vi "run conventional acq.vi"(8 "error in (no error)":errorcluster, 11 "Channel in":refnum<class "SPARC4_Channel.lvclass">) -> (0 "error out":errorcluster, 3 "Channel out":refnum<class "SPARC4_Channel.lvclass">)   [LabVIEW 2018, in "SPARC4_Channel.lvclass"]
doc: "Run the channel"
uses:
  SPARC4_Channel.lvclass
  C:/Users/Denis/Desktop/S4ACS/S4ACS/Channel/Channel.lvclass
  SPARC4_Channel.lvclass/SPARC4_Channel.ctl
  Channel/Channel.lvclass/Channel.ctl
  Sim_Ixon_Ultra/Sim_Ixon_Ultra.lvclass
  C:/Users/Denis/Desktop/S4ACS/S4ACS/Sim_CCD/Sim_CCD.lvclass
  State Machine/State Machine.lvclass
  Sim_CCD/Sim_CCD.lvclass
  RxTx/RxTx.lvclass
  Server/Server.lvclass
  Channel/Channel.lvclass
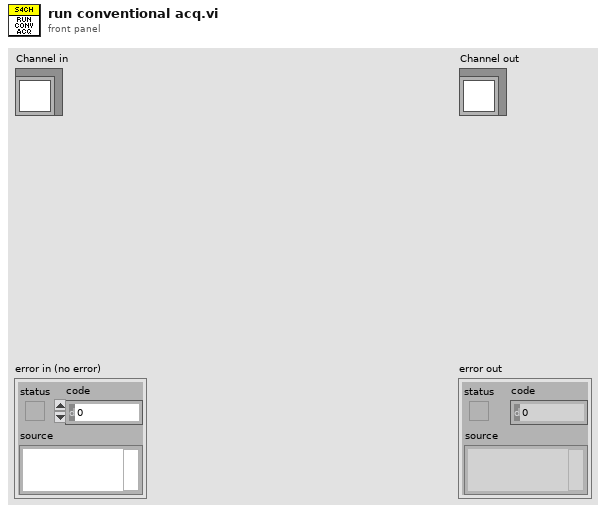
[diagram p1: front panel]
types:
  T1 = cluster{"State Machine.lvclass":refnum<class "State Machine.lvclass">, "RxTx.lvclass":refnum<class "RxTx.lvclass">, "Save_Header_RxTx.lvclass":refnum<class "RxTx.lvclass">, "Status SM.lvclass":refnum<class "State Machine.lvclass">, "Status RxTx.lvclass":refnum<class "RxTx.lvclass">, "servers array":refnum<class "Server.lvclass">[], "Events log file.lvclass":refnum<class "Log File.lvclass">, "Errors log file.lvclass":refnum<class "Log File.lvclass">, "Keywords log file.lvclass":refnum<class "Log File.lvclass">, "Sim_CCD.lvclass":refnum<class "Sim_CCD.lvclass">}
  T2 = typedef "LVDateTimeRec.ctl" = cluster{"fractional second":dbl, "second":i32, "minute":i32, "hour":i32, "day of month":i32, "month":i32, "year":i32, "day of week":i32, "day of year":i32, "DST":i32}
  T3 = cluster{"Time Acq Started":u32, "Image delay":u64, "Last update - CCD config":timestamp, "SYSTEMTIME":T2, "Readout time":dbl, "Time acq finished":u32, "effective exptime":dbl}
  T4 = cluster{"FRAMES_DONE":u16, "CCD_STATUS":string, "CURRENT_TEMPERATURE":i16, "TEMPERATURE_STATUS":string, "FRAME_EXPOSURE_TIME":dbl, "SERIAL_NUMBER":u16, "ACQUIRING":bool, "POWER":bool, "ACS MODE":bool}
  T5 = cluster{"Stop Acquisition":bool, "Abort Acquisition":bool, "Pause acquisition":bool, "wait expose command":bool, "video mode":bool, "stop app":bool}
  T6 = cluster{"CYCLES_DONE":u16, "LAST_IMAGE_NAME":string, "USED_DISK_SPACE":u16, "IMAGE_INDEX":u32, "acquisition error":bool}
  T7 = cluster{"EXPTIME":dbl, "#FRAMES":u32, "COOLER_POWER_STATUS":u16, "TEMP":i32}
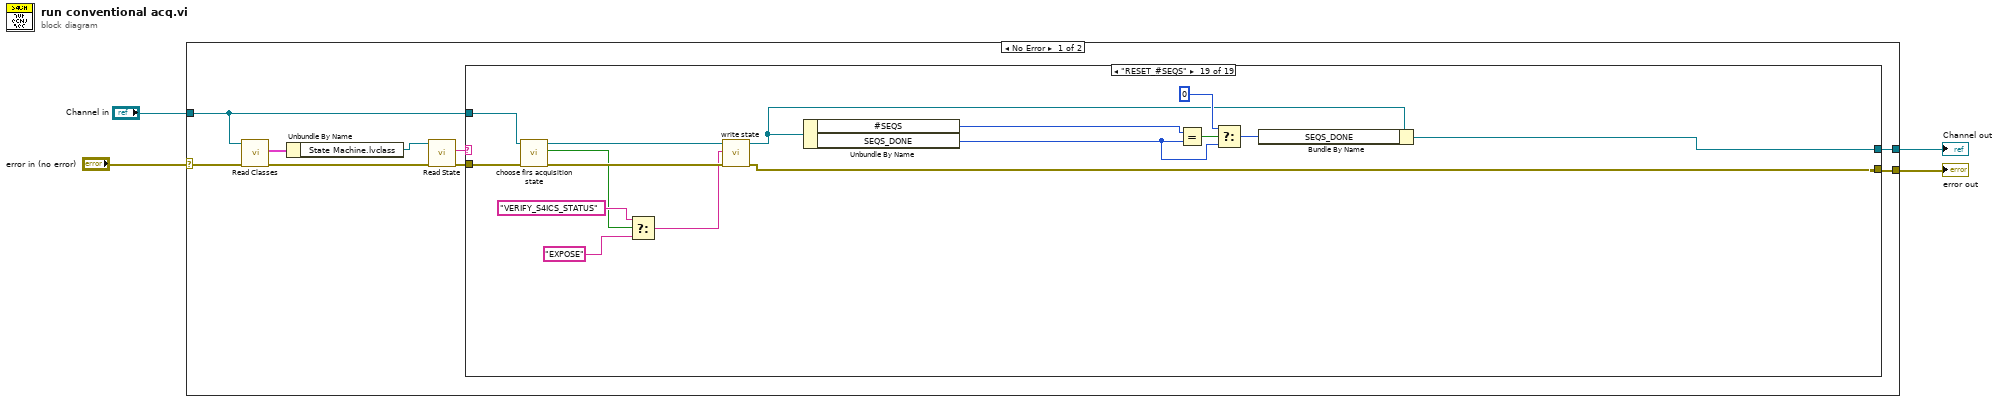
[diagram p0: block diagram]
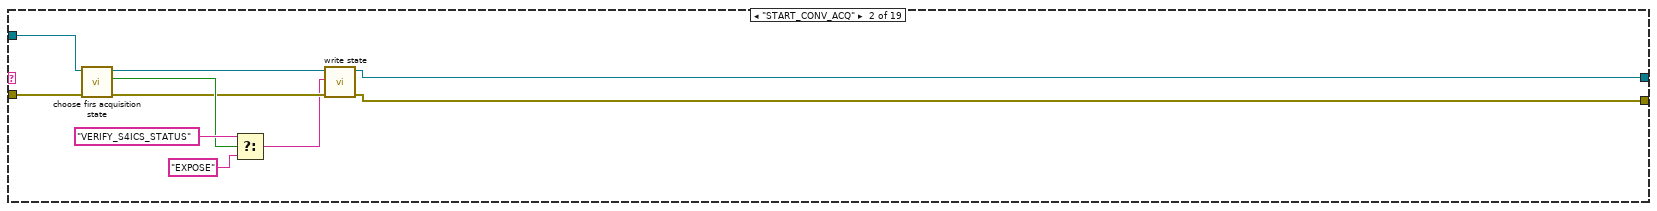
[diagram p3: hidden frame]
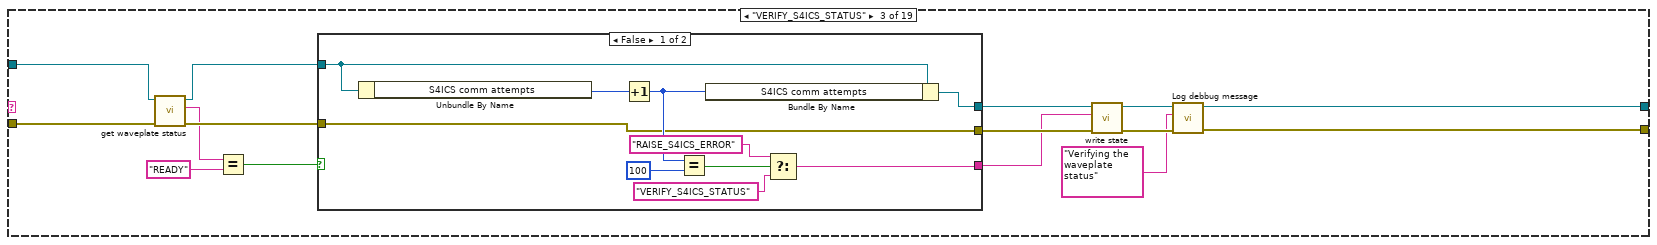
[diagram p4: hidden frame]
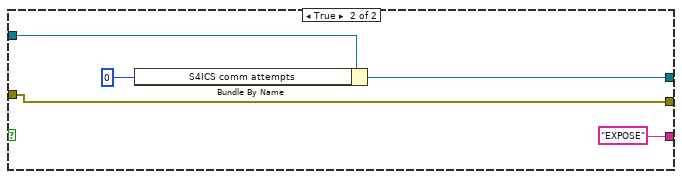
[diagram p5: hidden frame]
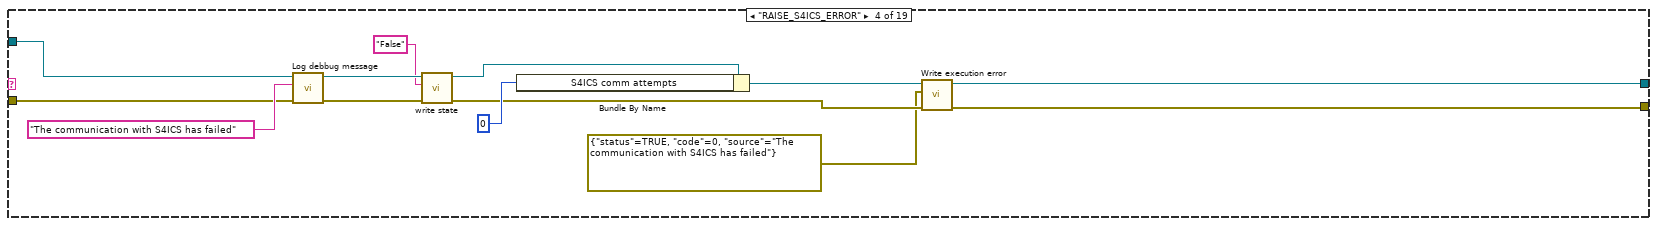
[diagram p6: hidden frame]
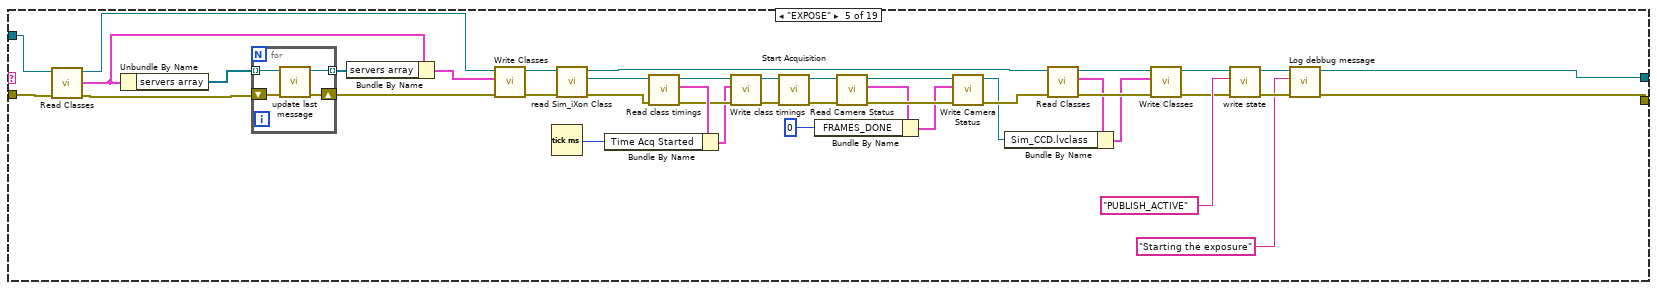
[diagram p7: hidden frame]
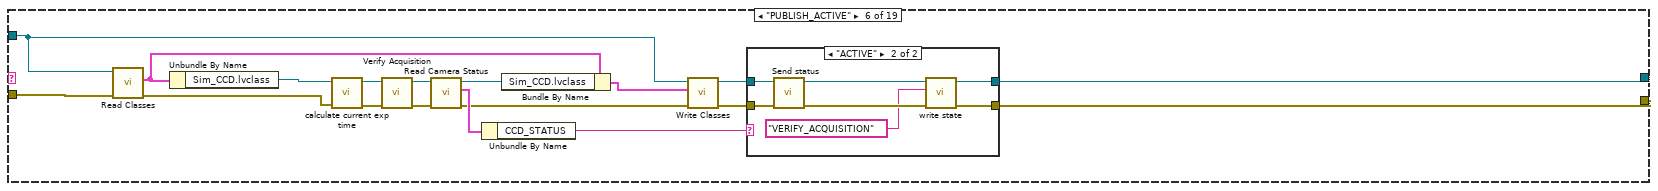
[diagram p8: hidden frame]
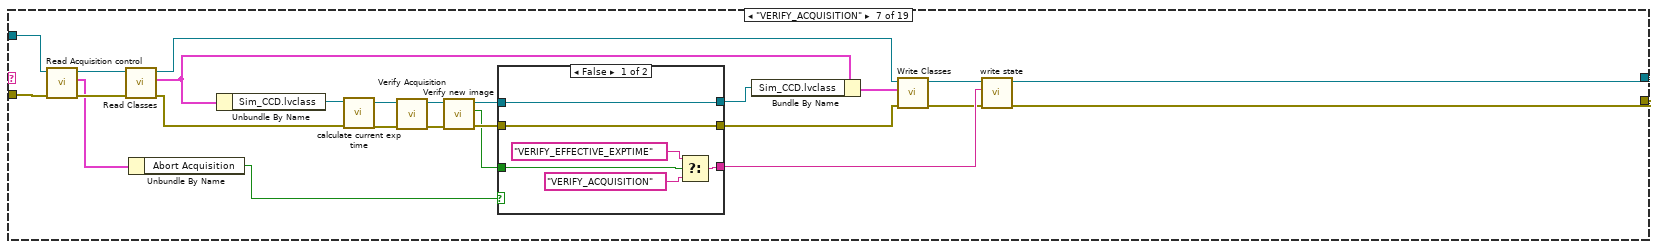
[diagram p10: hidden frame]
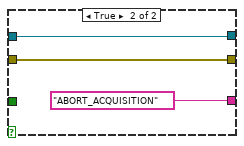
[diagram p11: hidden frame]
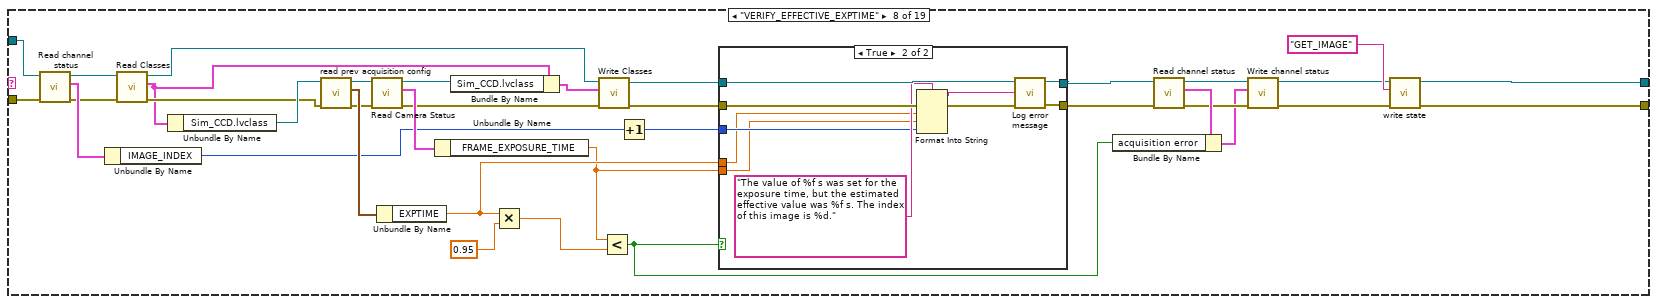
[diagram p12: hidden frame]
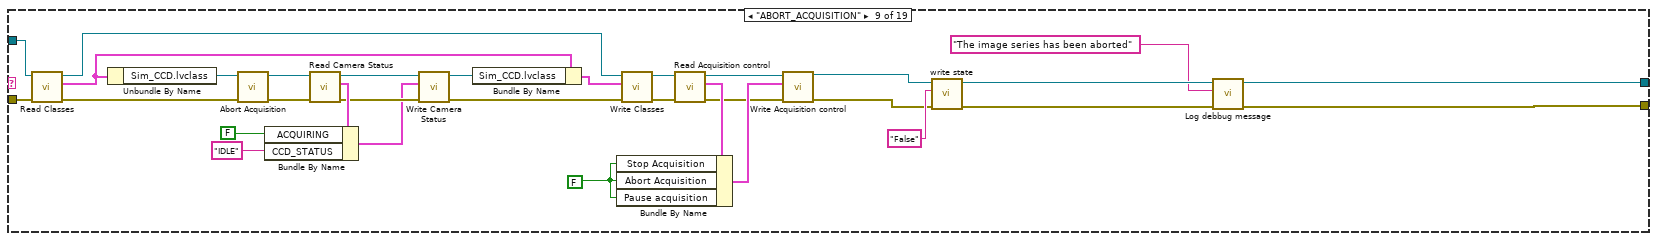
[diagram p14: hidden frame]
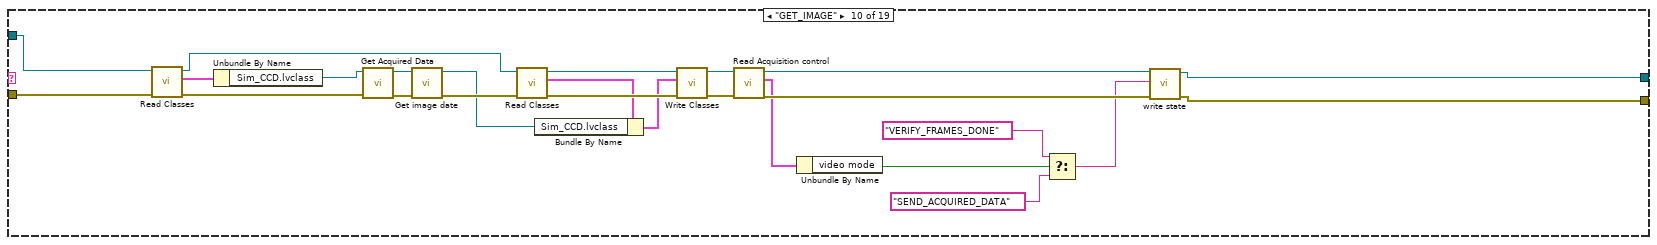
[diagram p15: hidden frame]
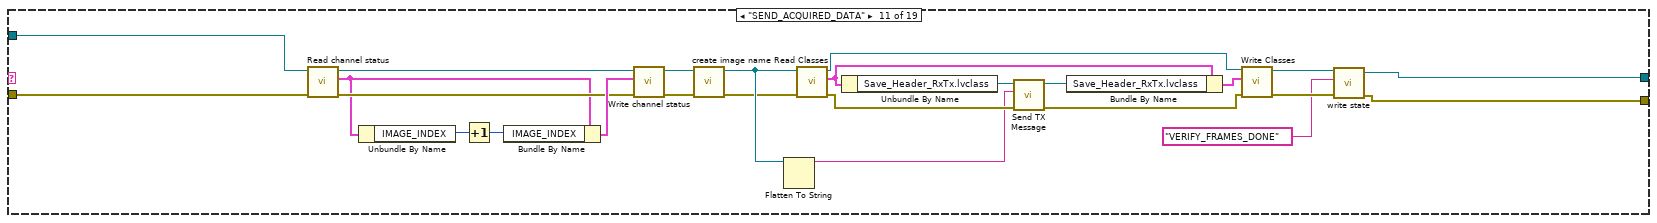
[diagram p16: hidden frame]
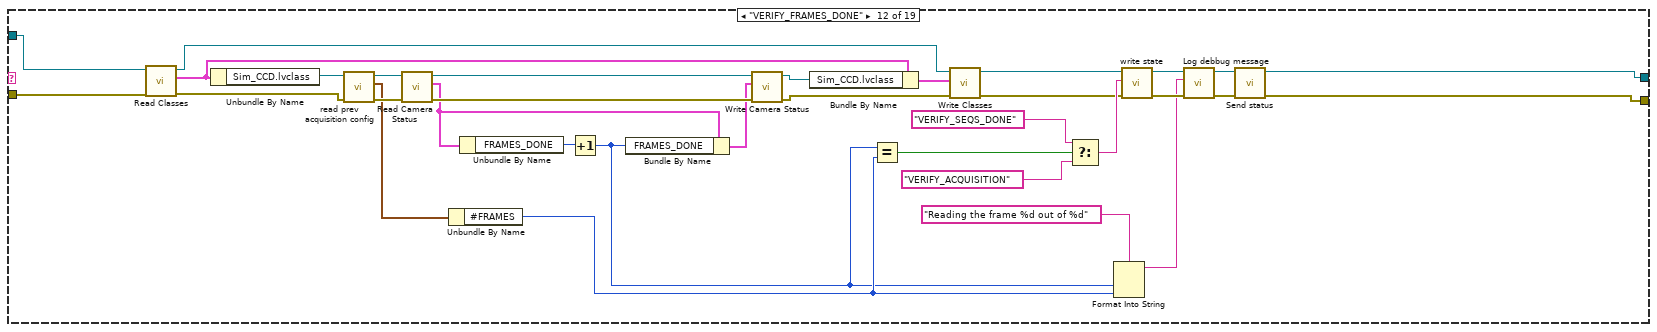
[diagram p17: hidden frame]
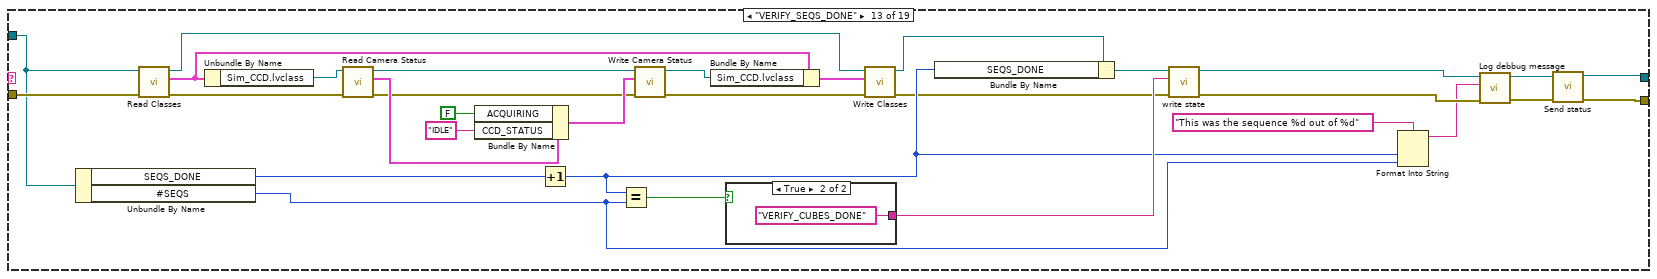
[diagram p18: hidden frame]
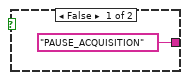
[diagram p19: hidden frame]
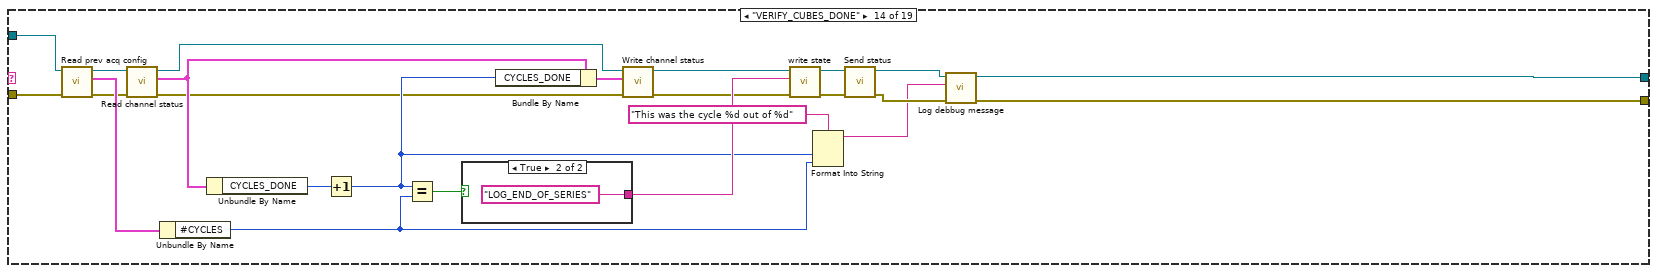
[diagram p20: hidden frame]
diagram:
  n1 = case shown="No Error" "error in (no error)" {
    selector: "error in (no error)" -> [w7 w486]
    tunnel: [w13 w486] -> w3
    tunnel: [w12 w485] -> w1
    tunnel: "Channel in" -> [w8 w485]
    frame No Error {
      n2 = call-dynamic "Read Classes.vi"("error in (no error)"=w7, "Channel in"=w8) -> ("error out"=w6:errorcluster, "Classes"=w9:T1)  [unwired: 7 in, 1 out]
      n3 = Unbundle By Name(w9) -> ("State Machine.lvclass"=w5:refnum<class "State Machine.lvclass">)
      n4 = call-dynamic "Read State.vi"("error in (no error)"=w6, "State Machine in"=w5) -> ("error out"=w11:errorcluster, "State"=w10:string)  [unwired: 7 in, 1 out]
      n5 = case shown="\"RESET_#SEQS\"" w10 {
        tunnel: w11 -> [w14 w22 w28 w66 w90 w124 w147 w188 w241 w275 w284 w328 w353 w378 w404 w408 w435 w460 w479]
        tunnel: [w14 w17 w34 w57 w100 w131 w163 w210 w244 w266 w304 w327 w340 w390 w400 w414 w438 w466 w481] -> w13
        tunnel: [w15 w18 w35 w58 w101 w132 w164 w211 w245 w265 w305 w326 w341 w389 w401 w413 w439 w465 w480] -> w12
        tunnel: w8 -> [w15 w21 w30 w67 w89 w119 w145 w182 w240 w276 w285 w329 w349 w376 w405 w409 w436 w461 w478]
        frame "False", Default {
        }
        frame "START_CONV_ACQ" {
          n6 = call "choose firs acquisition state.vi"("error in (no error)"=w22, "Channel in"=w21) -> ("error out"=w20:errorcluster, "verify S4ICS status"=w23:bool, "Channel out"=w19:refnum<class "SPARC4_Channel.lvclass">)  [unwired: 7 in]
          n7 = Select(t="VERIFY_S4ICS_STATUS" ("x"), s=w23, f="EXPOSE" ("x")) -> (s? t:f=w16:string)
          n8 = call "write state.vi"("error in (no error)"=w20, "state"=w16, "Channel in"=w19) -> ("error out"=w17:errorcluster, "Channel out"=w18:refnum<class "SPARC4_Channel.lvclass">)  [unwired: 7 in]
        }
        frame "VERIFY_S4ICS_STATUS" {
          n9 = call "get waveplate status.vi"("error in (no error)"=w28, "Channel in"=w30) -> ("error out"=w27:errorcluster, "wp condition"=w26:string, "Channel out"=w29:refnum<class "SPARC4_Channel.lvclass">)  [unwired: 7 in]
          n10 = Equal?(x=w26, y="READY") -> (x = y?=w39:bool)
          n11 = case shown="False" w39 {
            tunnel: w29 -> [w50 w55]
            tunnel: w27 -> [w43 w54]
            tunnel: [w42 w53] -> w38
            tunnel: [w43 w54] -> w37
            tunnel: [w41 "EXPOSE" ("y")] -> w36
            frame False {
              n12 = Unbundle By Name(w50) -> ("S4ICS comm attempts"=w49:u8)
              n13 = Increment(x=w49) -> (x+1=w48:u8)
              n14 = Equal?(x=w48, y=100) -> (x = y?=w46:bool)
              n15 = Bundle By Name(cluster=w50, "S4ICS comm attempts"=w48) -> (w42:refnum<class "SPARC4_Channel.lvclass">)
              n16 = Select(t="RAISE_S4ICS_ERROR" ("y"), s=w46, f="VERIFY_S4ICS_STATUS" ("y")) -> (s? t:f=w41:string)
            }
            frame True {
              n17 = Bundle By Name(cluster=w55, "S4ICS comm attempts"=u8 0) -> (w53:refnum<class "SPARC4_Channel.lvclass">)
            }
          }
          n18 = call "write state.vi"("error in (no error)"=w37, "state"=w36, "Channel in"=w38) -> ("error out"=w33:errorcluster, "Channel out"=w32:refnum<class "SPARC4_Channel.lvclass">)  [unwired: 7 in]
          n19 = call "Log debbug message.vi"("error in (no error)"=w33, "String"="Verifying the waveplate status" ("y"), "Channel in"=w32) -> ("error out"=w34:errorcluster, "Channel out"=w35:refnum<class "SPARC4_Channel.lvclass">)  [unwired: 7 in]
        }
        frame "RAISE_S4ICS_ERROR" {
          n20 = call "Log debbug message.vi"("error in (no error)"=w66, "String"="The communication with S4ICS has failed", "Channel in"=w67) -> ("error out"=w63:errorcluster, "Channel out"=w64:refnum<class "SPARC4_Channel.lvclass">)  [unwired: 7 in]
          n21 = call "write state.vi"("error in (no error)"=w63, "state"="False", "Channel in"=w64) -> ("error out"=w59:errorcluster, "Channel out"=w62:refnum<class "SPARC4_Channel.lvclass">)  [unwired: 7 in]
          n22 = Bundle By Name(cluster=w62, "S4ICS comm attempts"=u8 0) -> (w60:refnum<class "SPARC4_Channel.lvclass">)
          n23 = call-dynamic "Write execution error.vi"("error in (no error)"=w59, "execution error"=errorcluster {"status"=TRUE, "code"=0, "source"="The communication with S4ICS has failed"} ("error constant"), "Channel in"=w60) -> ("error out"=w57:errorcluster, "Channel out"=w58:refnum<class "SPARC4_Channel.lvclass">)  [unwired: 7 in]
        }
        frame "EXPOSE" {
          n24 = call-dynamic "Read Classes.vi"("error in (no error)"=w90, "Channel in"=w89) -> ("error out"=w86:errorcluster, "Classes"=w83:T1, "Channel out"=w87:refnum<class "SPARC4_Channel.lvclass">)  [unwired: 7 in]
          n25 = Unbundle By Name(w83) -> ("servers array"=w88:refnum<class "Server.lvclass">[])
          n26 = for {
            tunnel: w88 -> [w111] mode=indexing
            shift-right: [w114] -> w85
            shift-left: w86 -> [w112]
            tunnel: [w113] -> w82 mode=indexing
            n27 = call "update last message.vi"("error in (no error)"=w112, "Server in"=w111) -> ("error out"=w114:errorcluster, "Server out"=w113:refnum<class "Server.lvclass">)  [unwired: 8 in]
          }
          n28 = Bundle By Name(cluster=w83, "servers array"=w82) -> (w84:T1)
          n29 = call-dynamic "Write Classes.vi"("error in (no error)"=w85, "Classes"=w84, "Channel in"=w87) -> ("error out"=w79:errorcluster, "Channel out"=w80:refnum<class "SPARC4_Channel.lvclass">)  [unwired: 7 in]
          n30 = Tick Count (ms)() -> (millisecond timer value=w91:u32)
          n31 = call "read Sim_iXon Class.vi"("error in (no error)"=w79, "SPARC4_Channel in"=w80) -> ("error out"=w78:errorcluster, "Sim_Ixon_Ultra.lvclass"=w81:refnum<class "Sim_Ixon_Ultra.lvclass">, "SPARC4_Channel out"=w72:refnum<class "SPARC4_Channel.lvclass">)  [unwired: 7 in]
          n32 = call "Read class timings.vi"("error in (no error)"=w78, "Simulated Camera in"=w81) -> ("error out"=w94:errorcluster, "class timings"=w95:T3, "Simulated Camera out"=w93:refnum<class "Sim_Ixon_Ultra.lvclass">)  [unwired: 7 in]
          n33 = Bundle By Name(cluster=w95, "Time Acq Started"=w91) -> (w92:T3)
          n34 = call "Write class timings.vi"("error in (no error)"=w94, "class timings"=w92, "Simulated Camera in"=w93) -> ("error out"=w97:errorcluster, "Simulated Camera out"=w96:refnum<class "Sim_Ixon_Ultra.lvclass">)  [unwired: 7 in]
          n35 = call-dynamic "Start Acquisition.vi"("error in (no error)"=w97, "CCDCamera in"=w96) -> ("error out"=w103:errorcluster, "CCDCamera out"=w104:refnum<class "Sim_Ixon_Ultra.lvclass">)  [unwired: 8 in]
          n36 = call "Read Camera Status.vi"("error in (no error)"=w103, "CCDCamera in"=w104) -> ("error out"=w110:errorcluster, "camera status"=w108:T4, "CCDCamera out"=w109:refnum<class "Sim_Ixon_Ultra.lvclass">)  [unwired: 7 in]
          n37 = Bundle By Name(cluster=w108, "FRAMES_DONE"=u16 0) -> (w107:T4)
          n38 = call "Write Camera Status.vi"("error in (no error)"=w110, "camera status"=w107, "CCDCamera in"=w109) -> ("error out"=w77:errorcluster, "CCDCamera out"=w69:refnum<class "Sim_Ixon_Ultra.lvclass">)  [unwired: 7 in]
          n39 = call-dynamic "Read Classes.vi"("error in (no error)"=w77, "Channel in"=w72) -> ("error out"=w74:errorcluster, "Classes"=w71:T1, "Channel out"=w73:refnum<class "SPARC4_Channel.lvclass">)  [unwired: 7 in]
          n40 = Bundle By Name(cluster=w71, "Sim_CCD.lvclass"=w69) -> (w70:T1)
          n41 = call-dynamic "Write Classes.vi"("error in (no error)"=w74, "Classes"=w70, "Channel in"=w73) -> ("error out"=w76:errorcluster, "Channel out"=w75:refnum<class "SPARC4_Channel.lvclass">)  [unwired: 7 in]
          n42 = call "write state.vi"("error in (no error)"=w76, "state"="PUBLISH_ACTIVE", "Channel in"=w75) -> ("error out"=w99:errorcluster, "Channel out"=w102:refnum<class "SPARC4_Channel.lvclass">)  [unwired: 7 in]
          n43 = call "Log debbug message.vi"("error in (no error)"=w99, "String"="Starting the exposure", "Channel in"=w102) -> ("error out"=w100:errorcluster, "Channel out"=w101:refnum<class "SPARC4_Channel.lvclass">)  [unwired: 7 in]
        }
        frame "PUBLISH_ACTIVE" {
          n44 = call-dynamic "Read Classes.vi"("error in (no error)"=w124, "Channel in"=w119) -> ("error out"=w122:errorcluster, "Classes"=w117:T1)  [unwired: 7 in, 1 out]
          n45 = Unbundle By Name(w117) -> ("Sim_CCD.lvclass"=w123:refnum<class "Sim_CCD.lvclass">)
          n46 = call-dynamic "calculate current exp time.vi"("error in (no error)"=w122, "CCDCamera in"=w123) -> ("error out"=w125:errorcluster, "CCDCamera out"=w126:refnum<class "Sim_CCD.lvclass">)  [unwired: 8 in]
          n47 = call-dynamic "Verify Acquisition.vi"("error in (no error)"=w125, "CCDCamera in"=w126) -> ("error out"=w127:errorcluster, "CCDCamera out"=w128:refnum<class "Sim_CCD.lvclass">)  [unwired: 8 in]
          n48 = call "Read Camera Status.vi"("error in (no error)"=w127, "CCDCamera in"=w128) -> ("error out"=w118:errorcluster, "camera status"=w130:T4, "CCDCamera out"=w116:refnum<class "Sim_CCD.lvclass">)  [unwired: 7 in]
          n49 = Unbundle By Name(w130) -> ("CCD_STATUS"=w129:string)
          n50 = Bundle By Name(cluster=w117, "Sim_CCD.lvclass"=w116) -> (w115:T1)
          n51 = call-dynamic "Write Classes.vi"("error in (no error)"=w118, "Classes"=w115, "Channel in"=w119) -> ("error out"=w120:errorcluster, "Channel out"=w121:refnum<class "SPARC4_Channel.lvclass">)  [unwired: 7 in]
          n52 = case shown="\"ACTIVE\"" w129 {
            tunnel: w121 -> [w134 w137]
            tunnel: [w134 w141] -> w132
            tunnel: [w133 w140] -> w131
            tunnel: w120 -> [w133 w136]
            frame "False", Default {
            }
            frame "ACTIVE" {
              n53 = call-dynamic "Send status.vi"("error in (no error)"=w136, "Channel in"=w137) -> ("error out"=w139:errorcluster, "Channel out"=w138:refnum<class "SPARC4_Channel.lvclass">)  [unwired: 8 in]
              n54 = call "write state.vi"("error in (no error)"=w139, "state"="VERIFY_ACQUISITION", "Channel in"=w138) -> ("error out"=w140:errorcluster, "Channel out"=w141:refnum<class "SPARC4_Channel.lvclass">)  [unwired: 7 in]
            }
          }
        }
        frame "VERIFY_ACQUISITION" {
          n55 = call "Read Acquisition control.vi"("error in (no error)"=w147, "Channel in"=w145) -> ("error out"=w146:errorcluster, "Acquisition control"=w143:T5, "Channel out"=w144:refnum<class "SPARC4_Channel.lvclass">)  [unwired: 7 in]
          n56 = call-dynamic "Read Classes.vi"("error in (no error)"=w146, "Channel in"=w144) -> ("error out"=w153:errorcluster, "Classes"=w150:T1, "Channel out"=w152:refnum<class "SPARC4_Channel.lvclass">)  [unwired: 7 in]
          n57 = Unbundle By Name(w143) -> ("Abort Acquisition"=w142:bool)
          n58 = Unbundle By Name(w150) -> ("Sim_CCD.lvclass"=w151:refnum<class "Sim_CCD.lvclass">)
          n59 = call-dynamic "calculate current exp time.vi"("error in (no error)"=w153, "CCDCamera in"=w151) -> ("error out"=w159:errorcluster, "CCDCamera out"=w160:refnum<class "Sim_CCD.lvclass">)  [unwired: 8 in]
          n60 = call-dynamic "Verify Acquisition.vi"("error in (no error)"=w159, "CCDCamera in"=w160) -> ("error out"=w166:errorcluster, "CCDCamera out"=w165:refnum<class "Sim_CCD.lvclass">)  [unwired: 8 in]
          n61 = call-dynamic "Verify new image.vi"("error in (no error)"=w166, "CCDCamera in"=w165) -> ("error out"=w161:errorcluster, "New Images ?"=w157:bool, "CCDCamera out"=w162:refnum<class "Sim_CCD.lvclass">)  [unwired: 7 in]
          n62 = case shown="False" w142 {
            tunnel: w162 -> [w172 w175]
            tunnel: w161 -> [w171 w174]
            tunnel: [w172 w175] -> w148
            tunnel: [w171 w174] -> w154
            tunnel: [w168 "ABORT_ACQUISITION"] -> w158
            tunnel: w157 -> [w167 _]
            frame False {
              n63 = Select(t="VERIFY_EFFECTIVE_EXPTIME", s=w167, f="VERIFY_ACQUISITION") -> (s? t:f=w168:string)
            }
            frame True {
            }
          }
          n64 = Bundle By Name(cluster=w150, "Sim_CCD.lvclass"=w148) -> (w149:T1)
          n65 = call-dynamic "Write Classes.vi"("error in (no error)"=w154, "Classes"=w149, "Channel in"=w152) -> ("error out"=w156:errorcluster, "Channel out"=w155:refnum<class "SPARC4_Channel.lvclass">)  [unwired: 7 in]
          n66 = call "write state.vi"("error in (no error)"=w156, "state"=w158, "Channel in"=w155) -> ("error out"=w163:errorcluster, "Channel out"=w164:refnum<class "SPARC4_Channel.lvclass">)  [unwired: 7 in]
        }
        frame "VERIFY_EFFECTIVE_EXPTIME" {
          n67 = call-dynamic "Read channel status.vi"("error in (no error)"=w188, "Channel in"=w182) -> ("error out"=w187:errorcluster, "channel status"=w190:T6, "Channel out"=w186:refnum<class "SPARC4_Channel.lvclass">)  [unwired: 7 in]
          n68 = Unbundle By Name(w190) -> ("IMAGE_INDEX"=w189:u32)
          n69 = call-dynamic "Read Classes.vi"("error in (no error)"=w187, "Channel in"=w186) -> ("error out"=w184:errorcluster, "Classes"=w178:T1, "Channel out"=w181:refnum<class "SPARC4_Channel.lvclass">)  [unwired: 7 in]
          n70 = Unbundle By Name(w178) -> ("Sim_CCD.lvclass"=w185:refnum<class "Sim_CCD.lvclass">)
          n71 = call "read prev acquisition config.vi"("error in (no error)"=w184, "Simulated_CCD_Camera in"=w185) -> ("error out"=w204:errorcluster, "prev acquisition configuration"=w206:T7, "Simulated_CCD_Camera out"=w205:refnum<class "Sim_CCD.lvclass">)  [unwired: 7 in]
          n72 = call "Read Camera Status.vi"("error in (no error)"=w204, "CCDCamera in"=w205) -> ("error out"=w179:errorcluster, "camera status"=w203:T4, "CCDCamera out"=w176:refnum<class "Sim_CCD.lvclass">)  [unwired: 7 in]
          n73 = Unbundle By Name(w206) -> ("EXPTIME"=w201:dbl)
          n74 = Unbundle By Name(w203) -> ("FRAME_EXPOSURE_TIME"=w200:dbl)
          n75 = Bundle By Name(cluster=w178, "Sim_CCD.lvclass"=w176) -> (w177:T1)
          n76 = Multiply(x=w201, y=0.95) -> (x*y=w207:dbl)
          n77 = call-dynamic "Write Classes.vi"("error in (no error)"=w179, "Classes"=w177, "Channel in"=w181) -> ("error out"=w183:errorcluster, "Channel out"=w180:refnum<class "SPARC4_Channel.lvclass">)  [unwired: 7 in]
          n78 = Less?(x=w200, y=w207) -> (x < y?=w198:bool)
          n79 = Increment(x=w189) -> (x+1=w202:u32)
          n80 = case shown="True" w198 {
            tunnel: w180 -> [w213 w223]
            tunnel: [w213 w222] -> w197
            tunnel: [w212 w221] -> w196
            tunnel: w183 -> [w212 w220]
            tunnel: w202 -> [_ w216]
            tunnel: w201 -> [_ w215]
            tunnel: w200 -> [_ w214]
            frame False {
            }
            frame True {
              n81 = Format Into String(format string="The value of %f s was set for the exposure time, but the estimated effective value was %f s. The index of this image is %d.", error in=w220, w215, w214, w216) -> (resulting string=w217:string, error out=w219:errorcluster)  [unwired: 1 in]
              n82 = call "Log error message.vi"("error in (no error)"=w219, "String"=w217, "Channel in"=w223) -> ("error out"=w221:errorcluster, "Channel out"=w222:refnum<class "SPARC4_Channel.lvclass">)  [unwired: 7 in]
            }
          }
          n83 = call-dynamic "Read channel status.vi"("error in (no error)"=w196, "Channel in"=w197) -> ("error out"=w192:errorcluster, "channel status"=w199:T6, "Channel out"=w193:refnum<class "SPARC4_Channel.lvclass">)  [unwired: 7 in]
          n84 = Bundle By Name(cluster=w199, "acquisition error"=w198) -> (w191:T6)
          n85 = call-dynamic "Write channel status.vi"("error in (no error)"=w192, "channel status"=w191, "Channel in"=w193) -> ("error out"=w195:errorcluster, "Channel out"=w194:refnum<class "SPARC4_Channel.lvclass">)  [unwired: 7 in]
          n86 = call "write state.vi"("error in (no error)"=w195, "state"="GET_IMAGE", "Channel in"=w194) -> ("error out"=w210:errorcluster, "Channel out"=w211:refnum<class "SPARC4_Channel.lvclass">)  [unwired: 7 in]
        }
        frame "ABORT_ACQUISITION" {
          w224 = FALSE ("Acquiring")
          n87 = call-dynamic "Read Classes.vi"("error in (no error)"=w241, "Channel in"=w240) -> ("error out"=w238:errorcluster, "Classes"=w234:T1, "Channel out"=w233:refnum<class "SPARC4_Channel.lvclass">)  [unwired: 7 in]
          n88 = Unbundle By Name(w234) -> ("Sim_CCD.lvclass"=w239:refnum<class "Sim_CCD.lvclass">)
          n89 = call-dynamic "Abort Acquisition.vi"("error in (no error)"=w238, "CCDCamera in"=w239) -> ("error out"=w252:errorcluster, "CCDCamera out"=w253:refnum<class "Sim_CCD.lvclass">)  [unwired: 8 in]
          n90 = call "Read Camera Status.vi"("error in (no error)"=w252, "CCDCamera in"=w253) -> ("error out"=w250:errorcluster, "camera status"=w255:T4, "CCDCamera out"=w251:refnum<class "Sim_CCD.lvclass">)  [unwired: 7 in]
          n91 = Bundle By Name(cluster=w255, "ACQUIRING"=FALSE ("Acquiring"), "CCD_STATUS"="IDLE" ("STATUS")) -> (w249:T4)
          n92 = call "Write Camera Status.vi"("error in (no error)"=w250, "camera status"=w249, "CCDCamera in"=w251) -> ("error out"=w236:errorcluster, "CCDCamera out"=w237:refnum<class "Sim_CCD.lvclass">)  [unwired: 7 in]
          n93 = Bundle By Name(cluster=w234, "Sim_CCD.lvclass"=w237) -> (w235:T1)
          n94 = call-dynamic "Write Classes.vi"("error in (no error)"=w236, "Classes"=w235, "Channel in"=w233) -> ("error out"=w231:errorcluster, "Channel out"=w232:refnum<class "SPARC4_Channel.lvclass">)  [unwired: 7 in]
          n95 = call "Read Acquisition control.vi"("error in (no error)"=w231, "Channel in"=w232) -> ("error out"=w225:errorcluster, "Acquisition control"=w227:T5, "Channel out"=w230:refnum<class "SPARC4_Channel.lvclass">)  [unwired: 7 in]
          n96 = Bundle By Name(cluster=w227, "Stop Acquisition"=w224, "Abort Acquisition"=w224, "Pause acquisition"=w224) -> (w226:T5)
          n97 = call "Write Acquisition control.vi"("error in (no error)"=w225, "Acquisition control"=w226, "Channel in"=w230) -> ("error out"=w228:errorcluster, "Channel out"=w229:refnum<class "SPARC4_Channel.lvclass">)  [unwired: 7 in]
          n98 = call "write state.vi"("error in (no error)"=w228, "state"="False", "Channel in"=w229) -> ("error out"=w243:errorcluster, "Channel out"=w246:refnum<class "SPARC4_Channel.lvclass">)  [unwired: 7 in]
          n99 = call "Log debbug message.vi"("error in (no error)"=w243, "String"="The image series has been aborted", "Channel in"=w246) -> ("error out"=w244:errorcluster, "Channel out"=w245:refnum<class "SPARC4_Channel.lvclass">)  [unwired: 7 in]
        }
        frame "GET_IMAGE" {
          n100 = call-dynamic "Read Classes.vi"("error in (no error)"=w275, "Channel in"=w276) -> ("error out"=w273:errorcluster, "Classes"=w274:T1, "Channel out"=w271:refnum<class "SPARC4_Channel.lvclass">)  [unwired: 7 in]
          n101 = Unbundle By Name(w274) -> ("Sim_CCD.lvclass"=w272:refnum<class "Sim_CCD.lvclass">)
          n102 = call-dynamic "Get Acquired Data.vi"("error in (no error)"=w273, "CCDCamera in"=w272) -> ("error out"=w279:errorcluster, "CCDCamera out"=w280:refnum<class "Sim_CCD.lvclass">)  [unwired: 8 in]
          n103 = call-dynamic "Get image date.vi"("error in (no error)"=w279, "Simulated_CCD_Camera in"=w280) -> ("error out"=w278:errorcluster, "Simulated_CCD_Camera out"=w277:refnum<class "Sim_CCD.lvclass">)  [unwired: 8 in]
          n104 = call-dynamic "Read Classes.vi"("error in (no error)"=w278, "Channel in"=w271) -> ("error out"=w270:errorcluster, "Classes"=w269:T1, "Channel out"=w268:refnum<class "SPARC4_Channel.lvclass">)  [unwired: 7 in]
          n105 = Bundle By Name(cluster=w269, "Sim_CCD.lvclass"=w277) -> (w267:T1)
          n106 = call-dynamic "Write Classes.vi"("error in (no error)"=w270, "Classes"=w267, "Channel in"=w268) -> ("error out"=w263:errorcluster, "Channel out"=w264:refnum<class "SPARC4_Channel.lvclass">)  [unwired: 7 in]
          n107 = call "Read Acquisition control.vi"("error in (no error)"=w263, "Channel in"=w264) -> ("error out"=w261:errorcluster, "Acquisition control"=w260:T5, "Channel out"=w262:refnum<class "SPARC4_Channel.lvclass">)  [unwired: 7 in]
          n108 = Unbundle By Name(w260) -> ("video mode"=w259:bool)
          n109 = Select(t="VERIFY_FRAMES_DONE", s=w259, f="SEND_ACQUIRED_DATA") -> (s? t:f=w256:string)
          n110 = call "write state.vi"("error in (no error)"=w261, "state"=w256, "Channel in"=w262) -> ("error out"=w266:errorcluster, "Channel out"=w265:refnum<class "SPARC4_Channel.lvclass">)  [unwired: 7 in]
        }
        frame "SEND_ACQUIRED_DATA" {
          n111 = call-dynamic "Read channel status.vi"("error in (no error)"=w284, "Channel in"=w285) -> ("error out"=w291:errorcluster, "channel status"=w283:T6, "Channel out"=w290:refnum<class "SPARC4_Channel.lvclass">)  [unwired: 7 in]
          n112 = Unbundle By Name(w283) -> ("IMAGE_INDEX"=w282:u32)
          n113 = Increment(x=w282) -> (x+1=w281:u32)
          n114 = Bundle By Name(cluster=w283, "IMAGE_INDEX"=w281) -> (w292:T6)
          n115 = call-dynamic "Write channel status.vi"("error in (no error)"=w291, "channel status"=w292, "Channel in"=w290) -> ("error out"=w286:errorcluster, "Channel out"=w287:refnum<class "SPARC4_Channel.lvclass">)  [unwired: 7 in]
          n116 = call-dynamic "create image name.vi"("error in (no error)"=w286, "Channel in"=w287) -> ("error out"=w288:errorcluster, "Channel out"=w289:refnum<class "SPARC4_Channel.lvclass">)  [unwired: 8 in]
          n117 = Flatten To String(anything=w289) -> (data string=w294:string)  [unwired: 3 in, 2 out]
          n118 = call-dynamic "Read Classes.vi"("error in (no error)"=w288, "Channel in"=w289) -> ("error out"=w299:errorcluster, "Classes"=w298:T1, "Channel out"=w293:refnum<class "SPARC4_Channel.lvclass">)  [unwired: 7 in]
          n119 = Unbundle By Name(w298) -> ("Save_Header_RxTx.lvclass"=w300:refnum<class "RxTx.lvclass">)
          n120 = call "Send TX Message.vi"("error in (no error)"=w299, "message"=w294, "RxTx in"=w300) -> ("error out"=w295:errorcluster, "RxTx out"=w296:refnum<class "RxTx.lvclass">)  [unwired: 7 in]
          n121 = Bundle By Name(cluster=w298, "Save_Header_RxTx.lvclass"=w296) -> (w297:T1)
          n122 = call-dynamic "Write Classes.vi"("error in (no error)"=w295, "Classes"=w297, "Channel in"=w293) -> ("error out"=w303:errorcluster, "Channel out"=w302:refnum<class "SPARC4_Channel.lvclass">)  [unwired: 7 in]
          n123 = call "write state.vi"("error in (no error)"=w303, "state"="VERIFY_FRAMES_DONE", "Channel in"=w302) -> ("error out"=w304:errorcluster, "Channel out"=w305:refnum<class "SPARC4_Channel.lvclass">)  [unwired: 7 in]
        }
        frame "VERIFY_FRAMES_DONE" {
          n124 = call-dynamic "Read Classes.vi"("error in (no error)"=w328, "Channel in"=w329) -> ("error out"=w310:errorcluster, "Classes"=w331:T1, "Channel out"=w330:refnum<class "SPARC4_Channel.lvclass">)  [unwired: 7 in]
          n125 = Unbundle By Name(w331) -> ("Sim_CCD.lvclass"=w311:refnum<class "Sim_CCD.lvclass">)
          n126 = call "read prev acquisition config.vi"("error in (no error)"=w310, "Simulated_CCD_Camera in"=w311) -> ("error out"=w316:errorcluster, "prev acquisition configuration"=w314:T7, "Simulated_CCD_Camera out"=w315:refnum<class "Sim_CCD.lvclass">)  [unwired: 7 in]
          n127 = call "Read Camera Status.vi"("error in (no error)"=w316, "CCDCamera in"=w315) -> ("error out"=w321:errorcluster, "camera status"=w317:T4, "CCDCamera out"=w320:refnum<class "Sim_CCD.lvclass">)  [unwired: 7 in]
          n128 = Unbundle By Name(w314) -> ("#FRAMES"=w307:u32)
          n129 = Unbundle By Name(w317) -> ("FRAMES_DONE"=w319:u16)
          n130 = Increment(x=w319) -> (x+1=w306:u16)
          n131 = Bundle By Name(cluster=w317, "FRAMES_DONE"=w306) -> (w318:T4)
          n132 = call "Write Camera Status.vi"("error in (no error)"=w321, "camera status"=w318, "CCDCamera in"=w320) -> ("error out"=w308:errorcluster, "CCDCamera out"=w309:refnum<class "Sim_CCD.lvclass">)  [unwired: 7 in]
          n133 = Bundle By Name(cluster=w331, "Sim_CCD.lvclass"=w309) -> (w332:T1)
          n134 = Equal?(x=w306, y=w307) -> (x = y?=w338:bool)
          n135 = call-dynamic "Write Classes.vi"("error in (no error)"=w308, "Classes"=w332, "Channel in"=w330) -> ("error out"=w333:errorcluster, "Channel out"=w334:refnum<class "SPARC4_Channel.lvclass">)  [unwired: 7 in]
          n136 = Select(t="VERIFY_SEQS_DONE", s=w338, f="VERIFY_ACQUISITION") -> (s? t:f=w335:string)
          n137 = Format Into String(format string="Reading the frame %d out of %d", w306, w307) -> (resulting string=w312:string)  [unwired: 2 in, 1 out]
          n138 = call "write state.vi"("error in (no error)"=w333, "state"=w335, "Channel in"=w334) -> ("error out"=w322:errorcluster, "Channel out"=w325:refnum<class "SPARC4_Channel.lvclass">)  [unwired: 7 in]
          n139 = call "Log debbug message.vi"("error in (no error)"=w322, "String"=w312, "Channel in"=w325) -> ("error out"=w323:errorcluster, "Channel out"=w324:refnum<class "SPARC4_Channel.lvclass">)  [unwired: 7 in]
          n140 = call-dynamic "Send status.vi"("error in (no error)"=w323, "Channel in"=w324) -> ("error out"=w327:errorcluster, "Channel out"=w326:refnum<class "SPARC4_Channel.lvclass">)  [unwired: 8 in]
        }
        frame "VERIFY_SEQS_DONE" {
          n141 = Unbundle By Name(w349) -> ("SEQS_DONE"=w356:u16, "#SEQS"=w354:u32)
          n142 = call-dynamic "Read Classes.vi"("error in (no error)"=w353, "Channel in"=w349) -> ("error out"=w352:errorcluster, "Classes"=w345:T1, "Channel out"=w348:refnum<class "SPARC4_Channel.lvclass">)  [unwired: 7 in]
          n143 = Unbundle By Name(w345) -> ("Sim_CCD.lvclass"=w351:refnum<class "Sim_CCD.lvclass">)
          n144 = call "Read Camera Status.vi"("error in (no error)"=w352, "CCDCamera in"=w351) -> ("error out"=w365:errorcluster, "camera status"=w369:T4, "CCDCamera out"=w366:refnum<class "Sim_CCD.lvclass">)  [unwired: 7 in]
          n145 = Bundle By Name(cluster=w369, "ACQUIRING"=FALSE, "CCD_STATUS"="IDLE") -> (w368:T4)
          n146 = Increment(x=w356) -> (x+1=w355:u16)
          n147 = Equal?(x=w355, y=w354) -> (x = y?=w367:bool)
          n148 = call "Write Camera Status.vi"("error in (no error)"=w365, "camera status"=w368, "CCDCamera in"=w366) -> ("error out"=w346:errorcluster, "CCDCamera out"=w343:refnum<class "Sim_CCD.lvclass">)  [unwired: 7 in]
          n149 = Bundle By Name(cluster=w345, "Sim_CCD.lvclass"=w343) -> (w344:T1)
          n150 = case shown="True" w367 {
            tunnel: ["PAUSE_ACQUISITION" "VERIFY_CUBES_DONE"] -> w361
            frame False {
            }
            frame True {
            }
          }
          n151 = call-dynamic "Write Classes.vi"("error in (no error)"=w346, "Classes"=w344, "Channel in"=w348) -> ("error out"=w347:errorcluster, "Channel out"=w350:refnum<class "SPARC4_Channel.lvclass">)  [unwired: 7 in]
          n152 = Bundle By Name(cluster=w350, "SEQS_DONE"=w355) -> (w362:refnum<class "SPARC4_Channel.lvclass">)
          n153 = call "write state.vi"("error in (no error)"=w347, "state"=w361, "Channel in"=w362) -> ("error out"=w359:errorcluster, "Channel out"=w360:refnum<class "SPARC4_Channel.lvclass">)  [unwired: 7 in]
          n154 = Format Into String(format string="This was the sequence %d out of %d", w355, w354) -> (resulting string=w357:string)  [unwired: 2 in, 1 out]
          n155 = call "Log debbug message.vi"("error in (no error)"=w359, "String"=w357, "Channel in"=w360) -> ("error out"=w339:errorcluster, "Channel out"=w342:refnum<class "SPARC4_Channel.lvclass">)  [unwired: 7 in]
          n156 = call-dynamic "Send status.vi"("error in (no error)"=w339, "Channel in"=w342) -> ("error out"=w340:errorcluster, "Channel out"=w341:refnum<class "SPARC4_Channel.lvclass">)  [unwired: 8 in]
        }
        frame "VERIFY_CUBES_DONE" {
          n157 = call-dynamic "Read prev acq config.vi"("error in (no error)"=w378, "Channel in"=w376) -> ("error out"=w377:errorcluster, "prev acq config"=w384:cluster{"suffix":string, "#CYCLES":u32}, "Channel out"=w375:refnum<class "SPARC4_Channel.lvclass">)  [unwired: 7 in]
          n158 = call-dynamic "Read channel status.vi"("error in (no error)"=w377, "Channel in"=w375) -> ("error out"=w374:errorcluster, "channel status"=w381:T6, "Channel out"=w373:refnum<class "SPARC4_Channel.lvclass">)  [unwired: 7 in]
          n159 = Unbundle By Name(w384) -> ("#CYCLES"=w383:u32)
          n160 = Unbundle By Name(w381) -> ("CYCLES_DONE"=w385:u16)
          n161 = Increment(x=w385) -> (x+1=w380:u16)
          n162 = Equal?(x=w380, y=w383) -> (x = y?=w395:bool)
          n163 = case shown="True" w395 {
            tunnel: ["PAUSE_ACQUISITION" "LOG_END_OF_SERIES"] -> w392
            frame False {
            }
            frame True {
            }
          }
          n164 = Bundle By Name(cluster=w381, "CYCLES_DONE"=w380) -> (w379:T6)
          n165 = call-dynamic "Write channel status.vi"("error in (no error)"=w374, "channel status"=w379, "Channel in"=w373) -> ("error out"=w382:errorcluster, "Channel out"=w372:refnum<class "SPARC4_Channel.lvclass">)  [unwired: 7 in]
          n166 = call "write state.vi"("error in (no error)"=w382, "state"=w392, "Channel in"=w372) -> ("error out"=w393:errorcluster, "Channel out"=w394:refnum<class "SPARC4_Channel.lvclass">)  [unwired: 7 in]
          n167 = Format Into String(format string="This was the cycle %d out of %d", w380, w383) -> (resulting string=w387:string)  [unwired: 2 in, 1 out]
          n168 = call-dynamic "Send status.vi"("error in (no error)"=w393, "Channel in"=w394) -> ("error out"=w391:errorcluster, "Channel out"=w388:refnum<class "SPARC4_Channel.lvclass">)  [unwired: 8 in]
          n169 = call "Log debbug message.vi"("error in (no error)"=w391, "String"=w387, "Channel in"=w388) -> ("error out"=w390:errorcluster, "Channel out"=w389:refnum<class "SPARC4_Channel.lvclass">)  [unwired: 7 in]
        }
        frame "LOG_END_OF_SERIES" {
          n170 = call "write state.vi"("error in (no error)"=w404, "state"="False", "Channel in"=w405) -> ("error out"=w402:errorcluster, "Channel out"=w403:refnum<class "SPARC4_Channel.lvclass">)  [unwired: 7 in]
          n171 = call "Log info message.vi"("error in (no error)"=w402, "String"="The acquisition of the image series has been finished", "Channel in"=w403) -> ("error out"=w400:errorcluster, "Channel out"=w401:refnum<class "SPARC4_Channel.lvclass">)  [unwired: 7 in]
        }
        frame "PAUSE_ACQUISITION" {
          n172 = call "Read Acquisition control.vi"("error in (no error)"=w408, "Channel in"=w409) -> ("error out"=w407:errorcluster, "Acquisition control"=w411:T5, "Channel out"=w406:refnum<class "SPARC4_Channel.lvclass">)  [unwired: 7 in]
          n173 = Unbundle By Name(w411) -> ("Pause acquisition"=w410:bool)
          n174 = Select(t="PAUSE_ACQUISITION", s=w410, f="STOP_ACQUISITION") -> (s? t:f=w412:string)
          n175 = call "write state.vi"("error in (no error)"=w407, "state"=w412, "Channel in"=w406) -> ("error out"=w414:errorcluster, "Channel out"=w413:refnum<class "SPARC4_Channel.lvclass">)  [unwired: 7 in]
        }
        frame "STOP_ACQUISITION" {
          n176 = call "Read Acquisition control.vi"("error in (no error)"=w435, "Channel in"=w436) -> ("error out"=w434:errorcluster, "Acquisition control"=w433:T5, "Channel out"=w430:refnum<class "SPARC4_Channel.lvclass">)  [unwired: 7 in]
          n177 = Bundle By Name(cluster=w433, "Stop Acquisition"=FALSE) -> (w432:T5)
          n178 = Unbundle By Name(w433) -> ("Stop Acquisition"=w437:bool)
          n179 = call "Write Acquisition control.vi"("error in (no error)"=w434, "Acquisition control"=w432, "Channel in"=w430) -> ("error out"=w428:errorcluster, "Channel out"=w429:refnum<class "SPARC4_Channel.lvclass">)  [unwired: 7 in]
          n180 = Select(t="False", s=w437, f="WAIT_EXPOSE_COMMAND") -> (s? t:f=w440:string)
          n181 = call "write state.vi"("error in (no error)"=w428, "state"=w440, "Channel in"=w429) -> ("error out"=w427:errorcluster, "Channel out"=w426:refnum<class "SPARC4_Channel.lvclass">)  [unwired: 7 in]
          n182 = call-dynamic "Read Classes.vi"("error in (no error)"=w427, "Channel in"=w426) -> ("error out"=w424:errorcluster, "Classes"=w421:T1, "Channel out"=w420:refnum<class "SPARC4_Channel.lvclass">)  [unwired: 7 in]
          n183 = Not(x=w437) -> (.not. x?=w441:bool)
          n184 = Unbundle By Name(w421) -> ("Sim_CCD.lvclass"=w425:refnum<class "Sim_CCD.lvclass">)
          n185 = Select(t="WAITING_EXPOSE_COMMAND" ("CCD_STATUS"), s=w441, f="IDLE" ("CCD_STATUS")) -> (s? t:f=w444:string)
          n186 = call "Read Camera Status.vi"("error in (no error)"=w424, "CCDCamera in"=w425) -> ("error out"=w446:errorcluster, "camera status"=w448:T4, "CCDCamera out"=w445:refnum<class "Sim_CCD.lvclass">)  [unwired: 7 in]
          n187 = Bundle By Name(cluster=w448, "CCD_STATUS"=w444) -> (w447:T4)
          n188 = call "Write Camera Status.vi"("error in (no error)"=w446, "camera status"=w447, "CCDCamera in"=w445) -> ("error out"=w423:errorcluster, "CCDCamera out"=w419:refnum<class "Sim_CCD.lvclass">)  [unwired: 7 in]
          n189 = Bundle By Name(cluster=w421, "Sim_CCD.lvclass"=w419) -> (w422:T1)
          n190 = call-dynamic "Write Classes.vi"("error in (no error)"=w423, "Classes"=w422, "Channel in"=w420) -> ("error out"=w417:errorcluster, "Channel out"=w418:refnum<class "SPARC4_Channel.lvclass">)  [unwired: 7 in]
          n191 = case shown="True" w437 {
            tunnel: w418 -> [w452 w457]
            tunnel: [w452 w456] -> w439
            tunnel: [w451 w455] -> w438
            tunnel: w417 -> [w451 w454]
            frame False {
            }
            frame True {
              n192 = call "Log debbug message.vi"("error in (no error)"=w454, "String"="The acquisition has been stopped", "Channel in"=w457) -> ("error out"=w455:errorcluster, "Channel out"=w456:refnum<class "SPARC4_Channel.lvclass">)  [unwired: 7 in]
            }
          }
        }
        frame "WAIT_EXPOSE_COMMAND" {
          n193 = call "Read Acquisition control.vi"("error in (no error)"=w460, "Channel in"=w461) -> ("error out"=w458:errorcluster, "Acquisition control"=w463:T5, "Channel out"=w459:refnum<class "SPARC4_Channel.lvclass">)  [unwired: 7 in]
          n194 = Unbundle By Name(w463) -> ("wait expose command"=w462:bool)
          n195 = Select(t="STOP_ACQUISITION", s=w462, f="RESET_#SEQS") -> (s? t:f=w464:string)
          n196 = call "write state.vi"("error in (no error)"=w458, "state"=w464, "Channel in"=w459) -> ("error out"=w466:errorcluster, "Channel out"=w465:refnum<class "SPARC4_Channel.lvclass">)  [unwired: 7 in]
        }
        frame "RESET_#SEQS" {
          n197 = call "choose firs acquisition state.vi"("error in (no error)"=w479, "Channel in"=w478) -> ("error out"=w476:errorcluster, "verify S4ICS status"=w472:bool, "Channel out"=w477:refnum<class "SPARC4_Channel.lvclass">)  [unwired: 7 in]
          n198 = Select(t="VERIFY_S4ICS_STATUS", s=w472, f="EXPOSE") -> (s? t:f=w474:string)
          n199 = call "write state.vi"("error in (no error)"=w476, "state"=w474, "Channel in"=w477) -> ("error out"=w481:errorcluster, "Channel out"=w482:refnum<class "SPARC4_Channel.lvclass">)  [unwired: 7 in]
          n200 = Unbundle By Name(w482) -> ("#SEQS"=w470:u32, "SEQS_DONE"=w469:u16)
          n201 = Equal?(x=w470, y=w469) -> (x = y?=w484:bool)
          n202 = Select(t=0, s=w484, f=w469) -> (s? t:f=w471:i32)
          n203 = Bundle By Name(cluster=w482, "SEQS_DONE"=w471) -> (w480:refnum<class "SPARC4_Channel.lvclass">)
        }
      }
    }
    frame Error {
    }
  }
  "error out" <- w3
  "Channel out" <- w1
